vi "Center Text.vi"(8 "error in (no error)":errorcluster, 11 "SubPanel in":refnum<class "SubPanel.lvclass">) -> (0 "error out":errorcluster, 3 "SubPanel out":refnum<class "SubPanel.lvclass">)   [LabVIEW 2012, in "SubPanel.lvlib" / "SubPanel.lvclass"]
uses:
  SubPanel.lvclass
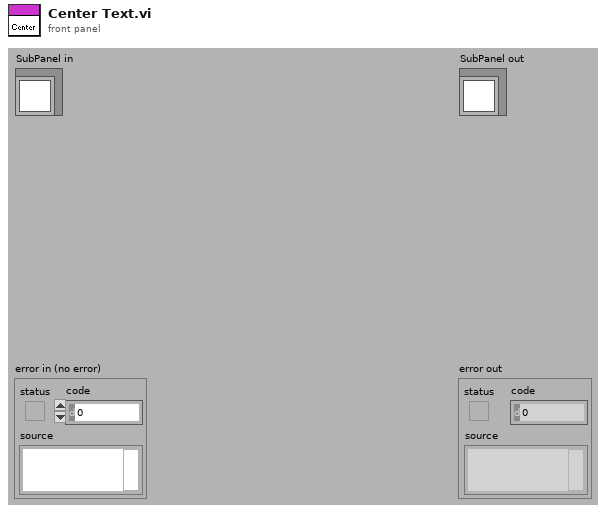
[diagram p1: front panel]
types:
  T1 = cluster{"left":i16, "top":i16, "right":i16, "bottom":i16}
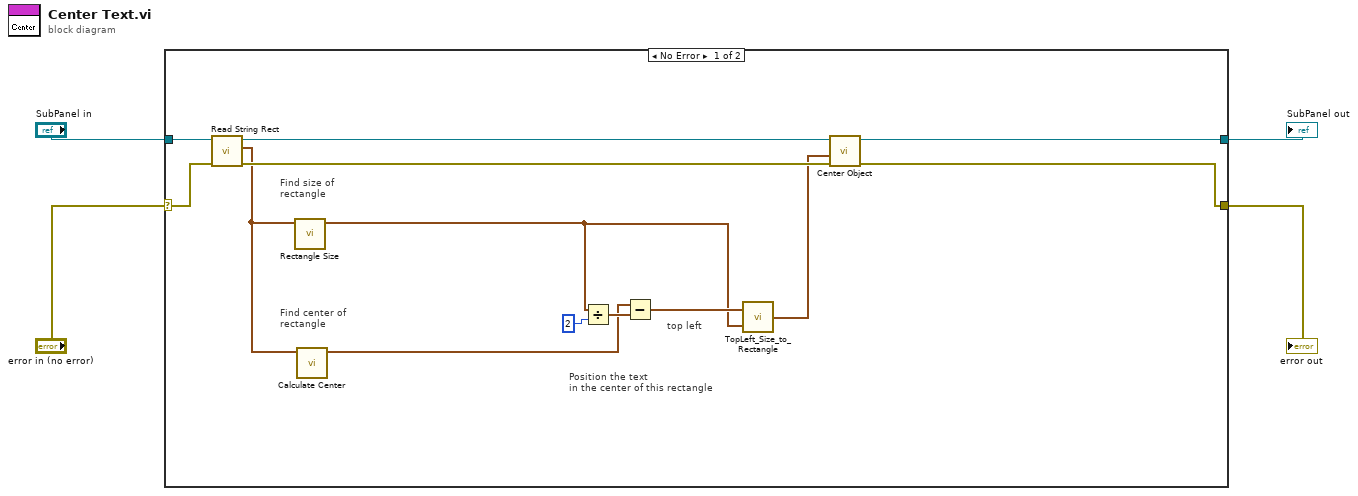
[diagram p0: block diagram]
diagram:
  n1 = case shown="No Error" "error in (no error)" {
    selector: "error in (no error)" -> [w13 w19]
    tunnel: [w5 w19] -> w1
    tunnel: [w6 w18] -> w2
    tunnel: "SubPanel in" -> [w14 w18]
    frame No Error {
      # "top left"
      # "Find size of\nrectangle"
      # "Position the text\nin the center of this rectangle"
      # "Find center of\nrectangle"
      n2 = call-dynamic "Read String Rect.vi"("error in (no error)"=w13, "Dialog.lvclass in"=w14) -> ("error out"=w9:errorcluster, "Object Rect"=w8:T1, "Dialog.lvclass out"=w10:refnum<class "SubPanel.lvclass">)  [unwired: 7 out]
      n3 = call "Rectangle Size.vi"("Rectangle"=w8) -> ("Rect Size"=w11:cluster{"width":i32, "height":i32})  [unwired: 10 out]
      n4 = call "Calculate Center.vi"("Rectangle"=w8) -> ("Center"=w16:cluster{"x":i32, "y":i32})  [unwired: 10 out]
      n5 = Divide(x=w11, y=2) -> (x/y=w17:cluster{"width":dbl, "height":dbl})
      n6 = Subtract(x=w16, y=w17) -> (x-y=w12:cluster{dbl, dbl})
      n7 = call "TopLeft_Size_to_Rectangle.vi"("Size"=w11, "Top Left"=w12) -> ("Rectangle"=w7:T1)
      n8 = call-dynamic "Center Object.vi"("error in"=w9, "Rectangle"=w7, "SubPanel in"=w10) -> ("error out"=w5:errorcluster, "SubPanel out"=w6:refnum<class "SubPanel.lvclass">)  [unwired: 1 in, 6 out]
    }
    frame Error {
    }
  }
  "error out" <- w1
  "SubPanel out" <- w2
